vi "LSCI332 GetResistance.vi"(11 "error in":errorcluster) -> (4 "Résistance":u16=50 caption="Résistance Chauffage", 15 "error out":errorcluster)   [LabVIEW 2019]
doc: "Ce Vi envoie à l'instrument la valeur de \"Manual output\" de chauffage désiré, en %."
uses:
  <vilib>/Utility/config.llb/Read Key (I32).vi
  <vilib>/Utility/config.llb/NI_LVConfig.lvlib
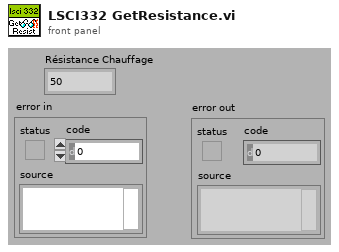
[diagram p1: front panel]
types:
  T1 = typedef "NI_LVConfig.lvlib/Config Data RefNum.ctl" = refnum<k1>
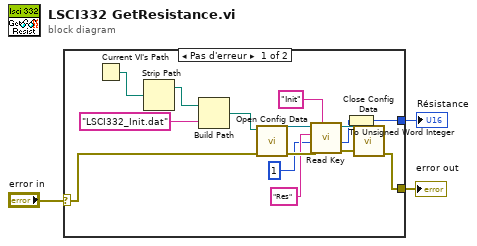
[diagram p0: block diagram]
diagram:
  n1 = case shown="Pas d'erreur" "error in" {
    selector: "error in" -> [w14 w19]
    tunnel: [w13 w19] -> w3
    tunnel: [w4 _] -> w1
    frame No Error {
      n2 = Current VI's Path() -> (path=w18:path)
      n3 = Strip Path(path=w18) -> (stripped path=w17:path)  [unwired: 1 out]
      n4 = Build Path(base path=w17, name or relative path="LSCI332_Init.dat") -> (appended path=w15:path)
      n5 = call <vilib>:"Open Config Data.vi"("error in (no error)"=w14, "configuration file path"=w15) -> ("error out"=w9:errorcluster, "refnum"=w10:T1)  [unwired: 7 in, 1 out]
      n6 = call-poly <vilib>:"Read Key.vi"("section"="Init", "error in (no error)"=w9, "default value"=1, "key"="Res", "refnum"=w10) -> ("error out"=w12:errorcluster, "value"=w5:i32, "refnum out"=w11:T1)  [unwired: 3 in, 1 out]
      n7 = To Unsigned Word Integer(number=w5) -> (unsigned 16bit integer=w4:u16)
      n8 = call <vilib>:"Close Config Data.vi"("error in (no error)"=w12, "refnum"=w11) -> ("error out"=w13:errorcluster)  [unwired: 8 in, 1 out]
    }
    frame Error {
    }
  }
  "error out" <- w3
  "Résistance" <- w1
